vi "Prepare Control.vi"(7 "VolatusAPI":refnum<class "VolatusAPI.lvclass">, 8 "error in (no error)":errorcluster, 11 "ValveControl in":refnum<class "HitAndHoldControl.lvclass">) -> (0 "error out":errorcluster, 3 "ValveControl out":refnum<class "HitAndHoldControl.lvclass">)   [LabVIEW 2020, in "VolatusControl.lvlib" / "HitAndHoldControl.lvclass"]
uses:
  HitAndHoldControl.lvclass
  Volatus/VolatusAPI/VolatusAPI.lvclass
  HitAndHoldControl.lvclass/HitAndHoldControl.ctl
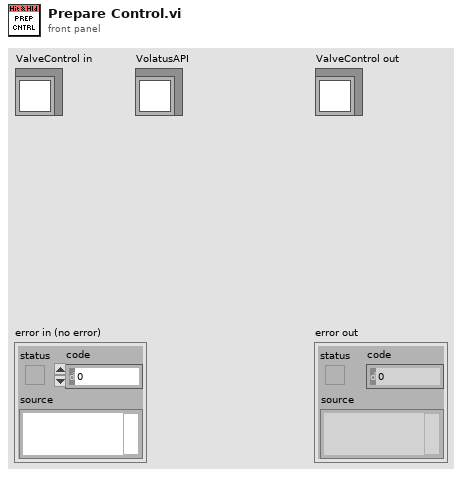
[diagram p1: front panel]
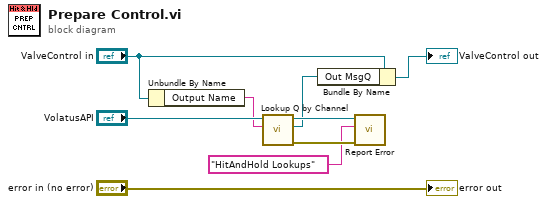
[diagram p0: block diagram]
diagram:
  n1 = Unbundle By Name("ValveControl in") -> ("Output Name"=w6:string)
  n2 = call "Lookup Q by Channel.vi"("Channel Name"=w6, "VolatusAPI in"="VolatusAPI") -> ("error out"=w2:errorcluster, "MessageQ"=w3:refnum<class "MessageQ.lvclass">, "VolatusAPI out"=w5:refnum<class "VolatusAPI.lvclass">)  [unwired: 7 in]
  n3 = Bundle By Name(cluster="ValveControl in", "Out MsgQ"=w3) -> (→"ValveControl out":refnum<class "HitAndHoldControl.lvclass">)
  n4 = call "Report Error.vi"("error in (no error)"=w2, "Context"="HitAndHold Lookups", "VolatusAPI in"=w5) -> ()  [unwired: 7 in, 2 out]
  "error out" <- "error in (no error)"
